vi "CheckOutLogic.vi"(7 "error in (no error)":errorcluster, 8 "Message Ref":refnum<vi>, 9 "Student ID":i32, 10 "Student List In":string[][](array[string])) -> (0 "error out":errorcluster, 1 "Total Elapsed Time":i32, 2 "Total Seconds Out":string, 3 "Elapsed Seconds":i32, 4 "Season Log ID":string, 5 "Record ID":string, 6 "Student List Size":i32)   [LabVIEW 2018]
doc: "Take current Hours, Minutes, Seconds, \nand Total Seconds, and add use to calculate \nthe difference between current time and the\n time at which the student checked in."
uses:
  Controls/SpreadsheetColumns.ctl
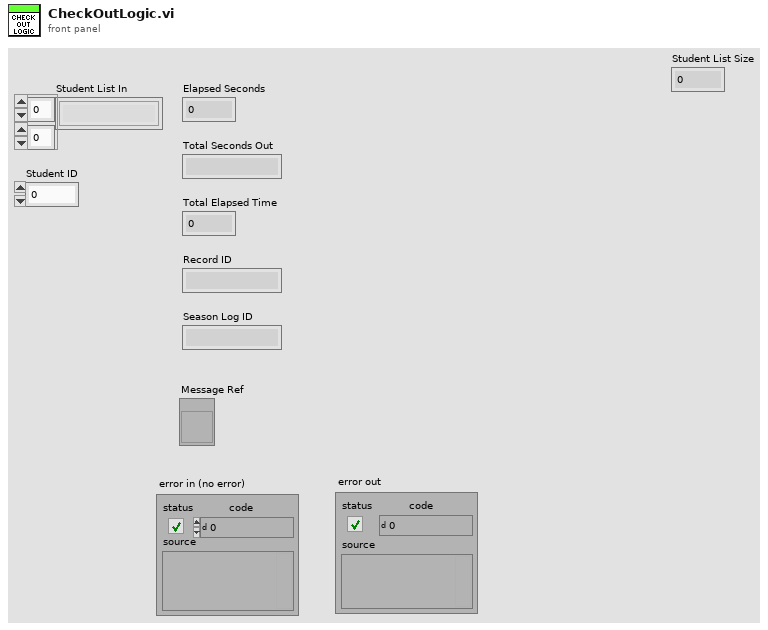
[diagram p1: front panel]
types:
  T1 = typedef "SpreadsheetColumns.ctl" = enum16{"Email", "CheckIn", "CheckOut", "Checkin Flag", "Hours", "Minutes", "Seconds", "Total Seconds", "Cat Points"}
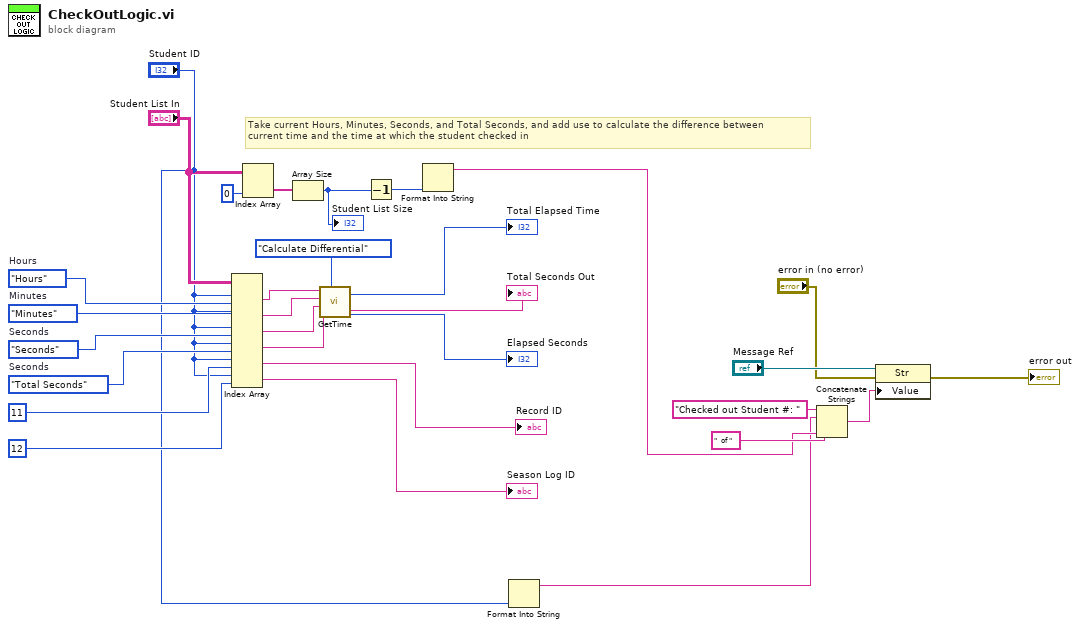
[diagram p0: block diagram]
diagram:
  w19 = SpreadsheetColumns."Total Seconds"  # Seconds
  w20 = SpreadsheetColumns."Seconds"  # Seconds
  w21 = SpreadsheetColumns."Minutes"  # Minutes
  w22 = SpreadsheetColumns."Hours"  # Hours
  # "Take current Hours, Minutes, Seconds, and Total Seconds, and add use to calculate the difference between\ncurrent time and the time at which the student checked in"
  n1 = Index Array(array="Student List In", index (row) #1="Student ID", index (col) #1=w22, index (row) #2="Student ID", index (col) #2=w21, index (row) #3="Student ID", index (col) #3=w20, index (row) #4="Student ID", index (col) #4=w19, index (row) #5="Student ID", index (col) #5=11 ("index (row)"), index (row) #6="Student ID", index (col) #6=12 ("disabled index (col)")) -> (element #1=w26:string, element #2=w27:string, element #3=w28:string, element #4=w25:string, element #5=→"Record ID":string, element #6=→"Season Log ID":string)
  n2 = Index Array(array="Student List In", index (col)=0 ("disabled index (col)")) -> (element=w10:string[])  [unwired: 1 in]
  n3 = Array Size(array=w10) -> (size(s)=w8:i32)
  "Student List Size" <- w8
  n4 = call "GetTime.vi"("State"=enum16{"Get Time", "Calculate Differential"}."Calculate Differential", "Total Seconds"=w25, "Stored Seconds"=w28, "Stored Minutes"=w27, "Stored Hours"=w26) -> ("Elapsed Seconds"=→"Elapsed Seconds":i32, "Total Seconds Out"=→"Total Seconds Out":string, "Total Elapsed Time"=→"Total Elapsed Time":i32)  [unwired: 1 in, 3 out]
  n5 = Decrement(x=w8) -> (x-1=w1:i32)
  n6 = Format Into String(w1) -> (resulting string=w7:string)  [unwired: 3 in, 1 out]
  n7 = Format Into String("Student ID") -> (resulting string=w2:string)  [unwired: 3 in, 1 out]
  n8 = Concatenate Strings("Checked out Student #: " ("string"), w2, "  of " ("string"), w7) -> (w6:string)
  n9 = property class="Str"(reference="Message Ref", error in="error in (no error)", "Value"=w6) -> (error out=→"error out":errorcluster)  [unwired: 1 out]
